vi "Auto Control.vi"   [LabVIEW 2018]
uses:
  <vilib>/Rock Robotics/Network Tables/NT Write String Array.vi
  SubSystems/Drive Train/Drive Train Global.vi
  Robot Global Data.vi
  SubSystems/Hatch Panel Intake/Hatch Panel Intake Global.vi
  SubSystems/Lift/Lift Global.vi
  SubSystems/Cargo Intake/Cargo Intake Global.vi
types:
  T1 = cluster{"X PID":cluster{"proportional gain (Kc)":dbl, "integral time (Ti, min)":dbl, "derivative time (Td, min)":dbl}, "Y PID":cluster{"proportional gain (Kc)":dbl, "integral time (Ti, min)":dbl, "derivative time (Td, min)":dbl}, "Z PID":cluster{"proportional gain (Kc)":dbl, "integral time (Ti, min)":dbl, "derivative time (Td, min)":dbl}}
  T2 = enum16{"Hatch Panel Zone 1", "Hatch Panel Zone 2", "Hatch Panel Zone 3", "Cargo Zone 1", "Cargo Zone 2", "Cargo Zone 3", "Cargo Ship Zone"}
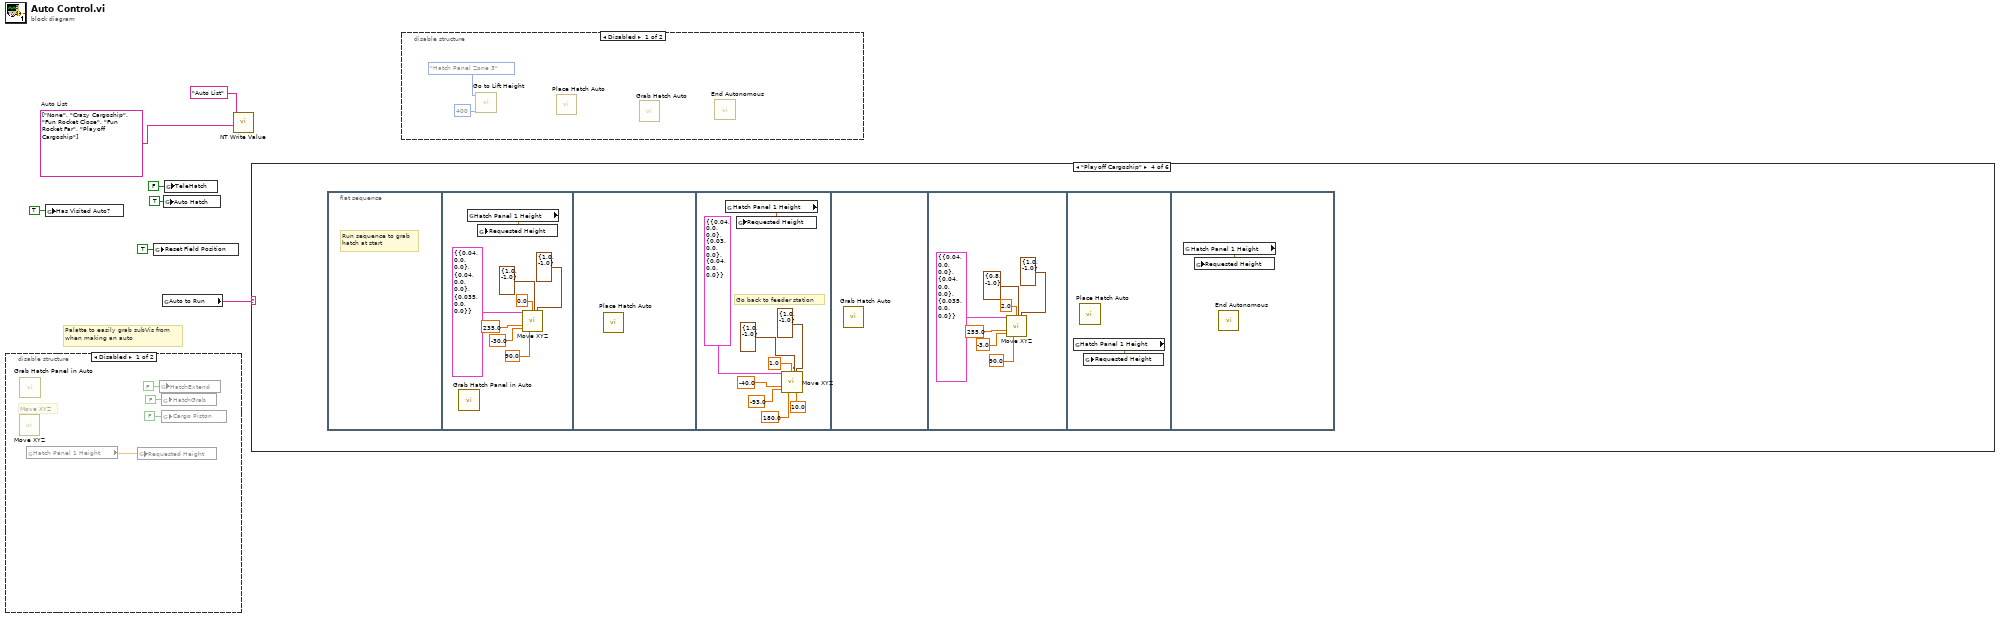
[diagram p0: block diagram]
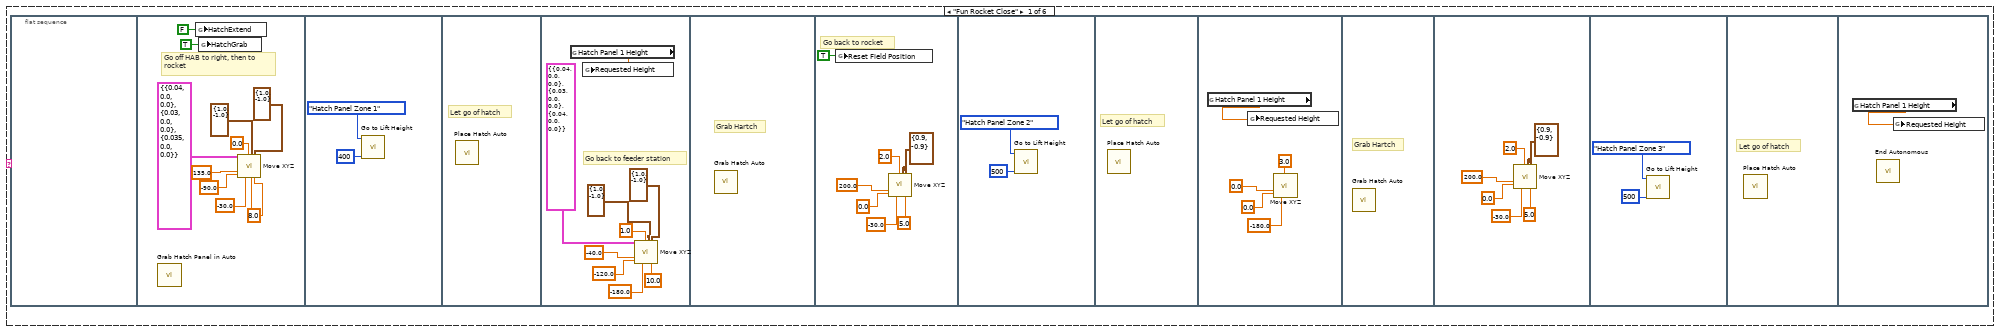
[diagram p4: hidden frame]
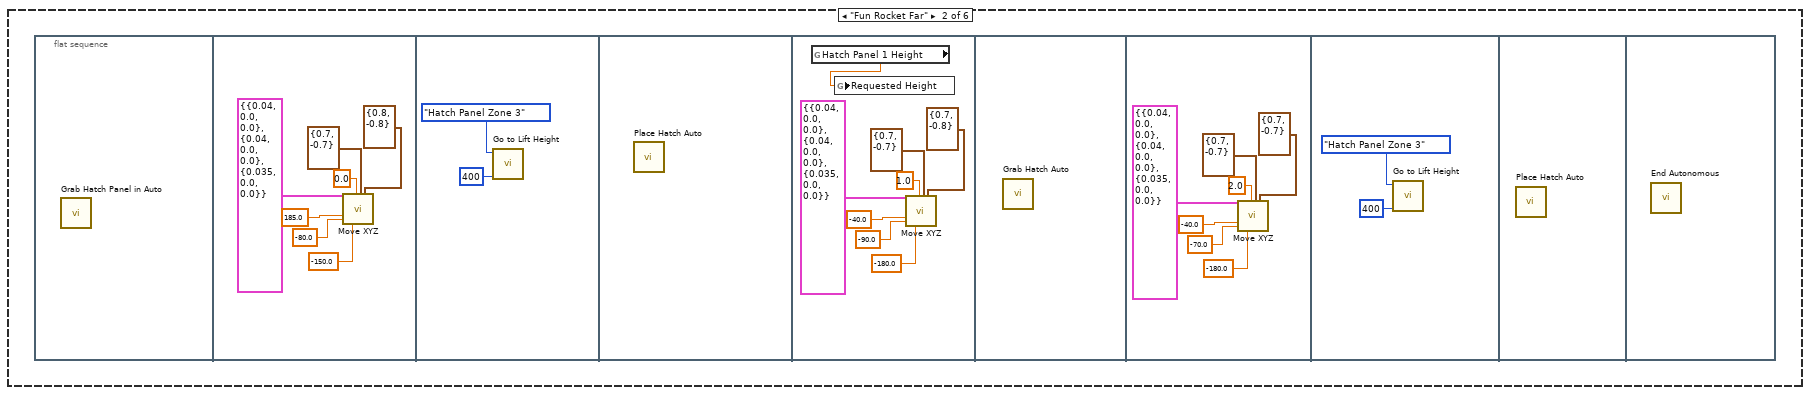
[diagram p5: hidden frame]
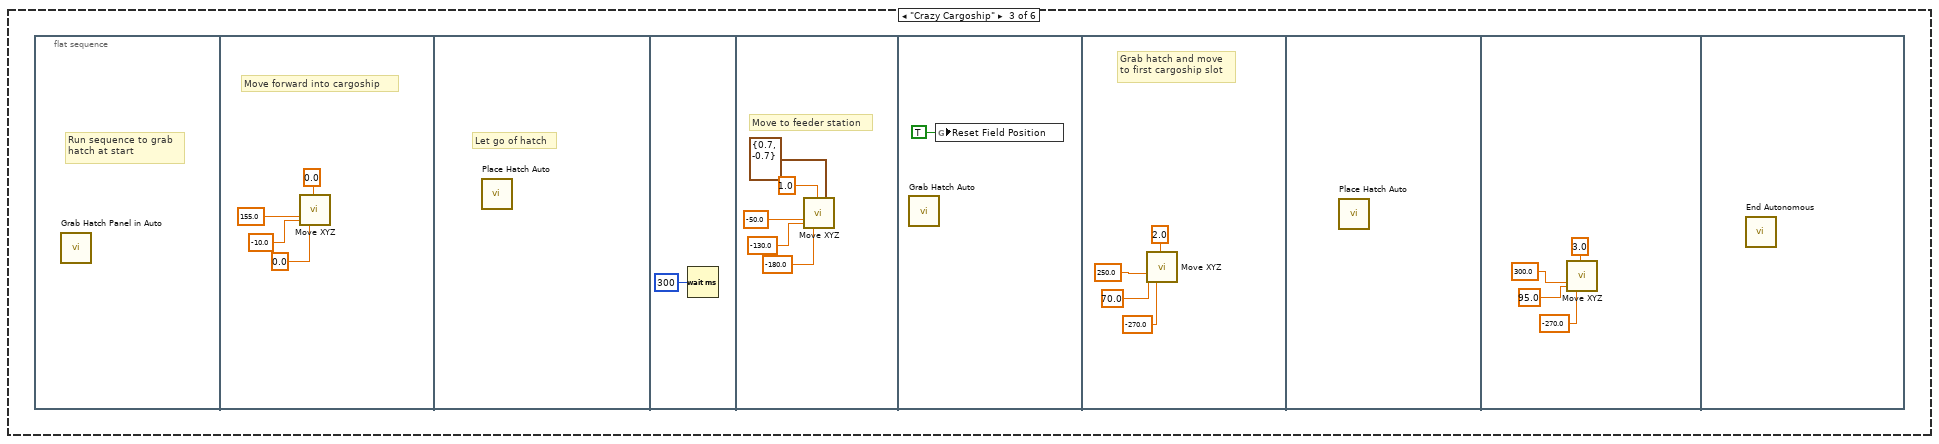
[diagram p6: hidden frame]
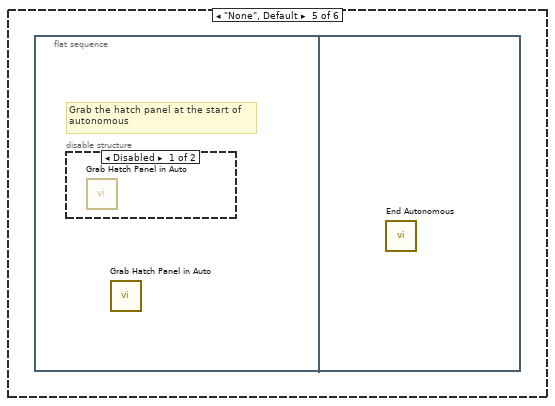
[diagram p7: hidden frame]
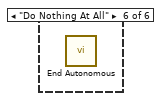
[diagram p9: hidden frame]
diagram:
  w6 = string[] ["None", "Crazy Cargoship", "Fun Rocket Close", "Fun Rocket Far", "Playoff Cargoship"]  # Auto List
  # "Palatte to easily grab subVis from\nwhen making an auto"
  n1 = disable-structure shown="Disabled" {
    frame Disabled {
      # "Move XYZ"
      n2 = call "Move XYZ.vi"() -> ()  [unwired: 28 in]
      n3 = call "Grab Hatch Panel in Auto.vi"() -> ()  [unwired: 12 in]
      n4 = global read "Lift Global.vi" "Hatch Panel 1 Height"() -> (w11:dbl)
      n5 = global write "Lift Global.vi" "Requested Height"(w11) -> ()
      n6 = global write "Hatch Panel Intake Global.vi" "HatchExtend"(FALSE ("HatchExtend")) -> ()
      n7 = global write "Hatch Panel Intake Global.vi" "HatchGrab"(FALSE ("HatchGrab")) -> ()
      n8 = global write "Cargo Intake Global.vi" "Cargo Piston"(FALSE ("Cargo Piston")) -> ()
    }
    frame Enabled {
    }
  }
  n9 = global write "Robot Global Data.vi" "Has Visited Auto?"(TRUE ("Has Visited Auto?")) -> ()
  n10 = global write "Drive Train Global.vi" "Reset Field Position"(TRUE ("Reset Field Position")) -> ()
  n11 = global read "Robot Global Data.vi" "Auto to Run"() -> (w5:string)
  n12 = global write "Hatch Panel Intake Global.vi" "Auto Hatch"(TRUE ("TeleHatch")) -> ()
  n13 = global write "Hatch Panel Intake Global.vi" "TeleHatch"(FALSE ("TeleHatch")) -> ()
  n14 = call-poly <vilib>:"NT Write Value.vi"("String Array"=w6, "Name"="Auto List") -> ()  [unwired: 9 in, 1 out]
  n15 = case shown="\"Playoff Cargoship\"" w5 {
    frame "Fun Rocket Close" {
      n16 = flat-sequence {
        frame #0 {
        }
        frame #1 {
          w15 = 8.0 ("X Stop Threshold")
          # "Go off HAB to right, then to\nrocket"
          n17 = call "Grab Hatch Panel in Auto.vi"() -> ()  [unwired: 12 in]
          n18 = global write "Hatch Panel Intake Global.vi" "HatchExtend"(FALSE ("HatchExtend")) -> ()
          n19 = global write "Hatch Panel Intake Global.vi" "HatchGrab"(TRUE ("HatchGrab")) -> ()
          n20 = call "Move XYZ.vi"("PID Gains In"=T1 {"X PID"={"proportional gain (Kc)"=0.04, "integral time (Ti, min)"=0.0, "derivative time (Td, min)"=0.0}, "Y PID"={"proportional gain (Kc)"=0.03, "integral time (Ti, min)"=0.0, "derivative time (Td, min)"=0.0}, "Z PID"={"proportional gain (Kc)"=0.035, "integral time (Ti, min)"=0.0, "derivative time (Td, min)"=0.0}}, "Y Target"=135.0, "X Target"=-90.0, "Gyro Target"=-30.0, "Movement"=0.0, "X Output Range"=cluster{"output high":dbl, "output low":dbl} {"output high"=1.0, "output low"=-1.0}, "X Stop Threshold"=w15, "Y Output Range"=cluster{"output high":dbl, "output low":dbl} {"output high"=1.0, "output low"=-1.0} ("X Output Range"), "Y Stop Threshold"=w15) -> ()  [unwired: 19 in]
        }
        frame #2 {
          n21 = call "Go to Lift Height.vi"("Time to Settle"=u32 400, "Lift Height to Go To"=T2."Hatch Panel Zone 1" ("y")) -> ()  [unwired: 10 in]
        }
        frame #3 {
          # "Let go of hatch"
          n22 = call "Place Hatch Auto.vi"() -> ()  [unwired: 12 in]
        }
        frame #4 {
          # "Go back to feeder station"
          n23 = global read "Lift Global.vi" "Hatch Panel 1 Height"() -> (w24:dbl)
          n24 = global write "Lift Global.vi" "Requested Height"(w24) -> ()
          n25 = call "Move XYZ.vi"("PID Gains In"=T1 {"X PID"={"proportional gain (Kc)"=0.04, "integral time (Ti, min)"=0.0, "derivative time (Td, min)"=0.0}, "Y PID"={"proportional gain (Kc)"=0.03, "integral time (Ti, min)"=0.0, "derivative time (Td, min)"=0.0}, "Z PID"={"proportional gain (Kc)"=0.04, "integral time (Ti, min)"=0.0, "derivative time (Td, min)"=0.0}}, "Y Target"=-40.0, "X Target"=-120.0, "Gyro Target"=-180.0, "Movement"=1.0, "X Output Range"=cluster{"output high":dbl, "output low":dbl} {"output high"=1.0, "output low"=-1.0}, "Y Output Range"=cluster{"output high":dbl, "output low":dbl} {"output high"=1.0, "output low"=-1.0} ("X Output Range"), "Y Stop Threshold"=10.0) -> ()  [unwired: 20 in]
        }
        frame #5 {
          # "Grab Hartch"
          n26 = call "Grab Hatch Auto.vi"() -> ()  [unwired: 12 in]
        }
        frame #6 {
          w33 = cluster{"output high":dbl, "output low":dbl} {"output high"=0.9, "output low"=-0.9} ("Y Output Range")
          # "Go back to rocket"
          n27 = global write "Drive Train Global.vi" "Reset Field Position"(TRUE ("Reset Field Position")) -> ()
          n28 = call "Move XYZ.vi"("Y Target"=200.0, "X Target"=0.0, "Gyro Target"=-30.0, "Movement"=2.0, "X Output Range"=w33, "Y Output Range"=w33, "Y Stop Threshold"=5.0) -> ()  [unwired: 21 in]
        }
        frame #7 {
          n29 = call "Go to Lift Height.vi"("Time to Settle"=u32 500, "Lift Height to Go To"=T2."Hatch Panel Zone 2" ("y")) -> ()  [unwired: 10 in]
        }
        frame #8 {
          # "Let go of hatch"
          n30 = call "Place Hatch Auto.vi"() -> ()  [unwired: 12 in]
        }
        frame #9 {
          n31 = global read "Lift Global.vi" "Hatch Panel 1 Height"() -> (w46:dbl)
          n32 = global write "Lift Global.vi" "Requested Height"(w46) -> ()
          n33 = call "Move XYZ.vi"("Y Target"=0.0, "X Target"=0.0, "Gyro Target"=-180.0, "Movement"=3.0) -> ()  [unwired: 24 in]
        }
        frame #10 {
          # "Grab Hartch"
          n34 = call "Grab Hatch Auto.vi"() -> ()  [unwired: 12 in]
        }
        frame #11 {
          w47 = cluster{"output high":dbl, "output low":dbl} {"output high"=0.9, "output low"=-0.9} ("Y Output Range")
          n35 = call "Move XYZ.vi"("Y Target"=200.0, "X Target"=0.0, "Gyro Target"=-30.0, "Movement"=2.0, "X Output Range"=w47, "Y Output Range"=w47, "Y Stop Threshold"=5.0) -> ()  [unwired: 21 in]
        }
        frame #12 {
          n36 = call "Go to Lift Height.vi"("Time to Settle"=u32 500, "Lift Height to Go To"=T2."Hatch Panel Zone 3" ("y")) -> ()  [unwired: 10 in]
        }
        frame #13 {
          # "Let go of hatch"
          n37 = call "Place Hatch Auto.vi"() -> ()  [unwired: 12 in]
        }
        frame #14 {
          n38 = global read "Lift Global.vi" "Hatch Panel 1 Height"() -> (w55:dbl)
          n39 = call "End Autonomous.vi"() -> ()  [unwired: 12 in]
          n40 = global write "Lift Global.vi" "Requested Height"(w55) -> ()
        }
      }
    }
    frame "Fun Rocket Far" {
      n41 = flat-sequence {
        frame #0 {
          n42 = call "Grab Hatch Panel in Auto.vi"() -> ()  [unwired: 12 in]
        }
        frame #1 {
          n43 = call "Move XYZ.vi"("PID Gains In"=T1 {"X PID"={"proportional gain (Kc)"=0.04, "integral time (Ti, min)"=0.0, "derivative time (Td, min)"=0.0}, "Y PID"={"proportional gain (Kc)"=0.04, "integral time (Ti, min)"=0.0, "derivative time (Td, min)"=0.0}, "Z PID"={"proportional gain (Kc)"=0.035, "integral time (Ti, min)"=0.0, "derivative time (Td, min)"=0.0}}, "Y Target"=185.0, "X Target"=-80.0, "Gyro Target"=-150.0, "Movement"=0.0, "X Output Range"=cluster{"output high":dbl, "output low":dbl} {"output high"=0.7, "output low"=-0.7}, "Y Output Range"=cluster{"output high":dbl, "output low":dbl} {"output high"=0.8, "output low"=-0.8} ("X Output Range")) -> ()  [unwired: 21 in]
        }
        frame #2 {
          n44 = call "Go to Lift Height.vi"("Time to Settle"=u32 400, "Lift Height to Go To"=T2."Hatch Panel Zone 3" ("y")) -> ()  [unwired: 10 in]
        }
        frame #3 {
          n45 = call "Place Hatch Auto.vi"() -> ()  [unwired: 12 in]
        }
        frame #4 {
          n46 = global read "Lift Global.vi" "Hatch Panel 1 Height"() -> (w65:dbl)
          n47 = global write "Lift Global.vi" "Requested Height"(w65) -> ()
          n48 = call "Move XYZ.vi"("PID Gains In"=T1 {"X PID"={"proportional gain (Kc)"=0.04, "integral time (Ti, min)"=0.0, "derivative time (Td, min)"=0.0}, "Y PID"={"proportional gain (Kc)"=0.04, "integral time (Ti, min)"=0.0, "derivative time (Td, min)"=0.0}, "Z PID"={"proportional gain (Kc)"=0.035, "integral time (Ti, min)"=0.0, "derivative time (Td, min)"=0.0}}, "Y Target"=-40.0, "X Target"=-90.0, "Gyro Target"=-180.0, "Movement"=1.0, "X Output Range"=cluster{"output high":dbl, "output low":dbl} {"output high"=0.7, "output low"=-0.7}, "Y Output Range"=cluster{"output high":dbl, "output low":dbl} {"output high"=0.7, "output low"=-0.8} ("X Output Range")) -> ()  [unwired: 21 in]
        }
        frame #5 {
          n49 = call "Grab Hatch Auto.vi"() -> ()  [unwired: 12 in]
        }
        frame #6 {
          n50 = call "Move XYZ.vi"("PID Gains In"=T1 {"X PID"={"proportional gain (Kc)"=0.04, "integral time (Ti, min)"=0.0, "derivative time (Td, min)"=0.0}, "Y PID"={"proportional gain (Kc)"=0.04, "integral time (Ti, min)"=0.0, "derivative time (Td, min)"=0.0}, "Z PID"={"proportional gain (Kc)"=0.035, "integral time (Ti, min)"=0.0, "derivative time (Td, min)"=0.0}}, "Y Target"=-40.0, "X Target"=-70.0, "Gyro Target"=-180.0, "Movement"=2.0, "X Output Range"=cluster{"output high":dbl, "output low":dbl} {"output high"=0.7, "output low"=-0.7}, "Y Output Range"=cluster{"output high":dbl, "output low":dbl} {"output high"=0.7, "output low"=-0.7} ("X Output Range")) -> ()  [unwired: 21 in]
        }
        frame #7 {
          n51 = call "Go to Lift Height.vi"("Time to Settle"=u32 400, "Lift Height to Go To"=T2."Hatch Panel Zone 3" ("y")) -> ()  [unwired: 10 in]
        }
        frame #8 {
          n52 = call "Place Hatch Auto.vi"() -> ()  [unwired: 12 in]
        }
        frame #9 {
          n53 = call "End Autonomous.vi"() -> ()  [unwired: 12 in]
        }
      }
    }
    frame "Crazy Cargoship" {
      n54 = flat-sequence {
        frame #0 {
          # "Run sequence to grab\nhatch at start"
          n55 = call "Grab Hatch Panel in Auto.vi"() -> ()  [unwired: 12 in]
        }
        frame #1 {
          # "Move forward into cargoship"
          n56 = call "Move XYZ.vi"("Y Target"=155.0, "X Target"=-10.0, "Gyro Target"=0.0, "Movement"=0.0) -> ()  [unwired: 24 in]
        }
        frame #2 {
          # "Let go of hatch"
          n57 = call "Place Hatch Auto.vi"() -> ()  [unwired: 12 in]
        }
        frame #3 {
          n58 = Wait (ms)(milliseconds to wait=u32 300) -> ()  [unwired: 1 out]
        }
        frame #4 {
          # "Move to feeder station"
          n59 = call "Move XYZ.vi"("Y Target"=-50.0, "X Target"=-130.0, "Gyro Target"=-180.0, "Movement"=1.0, "Y Output Range"=cluster{"output high":dbl, "output low":dbl} {"output high"=0.7, "output low"=-0.7}) -> ()  [unwired: 23 in]
        }
        frame #5 {
          n60 = call "Grab Hatch Auto.vi"() -> ()  [unwired: 12 in]
          n61 = global write "Drive Train Global.vi" "Reset Field Position"(TRUE ("Reset Field Position")) -> ()
        }
        frame #6 {
          # "Grab hatch and move\nto first cargoship slot"
          n62 = call "Move XYZ.vi"("Y Target"=250.0, "X Target"=70.0, "Gyro Target"=-270.0, "Movement"=2.0) -> ()  [unwired: 24 in]
        }
        frame #7 {
          n63 = call "Place Hatch Auto.vi"() -> ()  [unwired: 12 in]
        }
        frame #8 {
          n64 = call "Move XYZ.vi"("Y Target"=300.0, "X Target"=95.0, "Gyro Target"=-270.0, "Movement"=3.0) -> ()  [unwired: 24 in]
        }
        frame #9 {
          n65 = call "End Autonomous.vi"() -> ()  [unwired: 12 in]
        }
      }
    }
    frame "Playoff Cargoship" {
      n66 = flat-sequence {
        frame #0 {
          # "Run sequence to grab\nhatch at start"
        }
        frame #1 {
          n67 = call "Grab Hatch Panel in Auto.vi"() -> ()  [unwired: 12 in]
          n68 = global read "Lift Global.vi" "Hatch Panel 1 Height"() -> (w101:dbl)
          n69 = global write "Lift Global.vi" "Requested Height"(w101) -> ()
          n70 = call "Move XYZ.vi"("PID Gains In"=T1 {"X PID"={"proportional gain (Kc)"=0.04, "integral time (Ti, min)"=0.0, "derivative time (Td, min)"=0.0}, "Y PID"={"proportional gain (Kc)"=0.04, "integral time (Ti, min)"=0.0, "derivative time (Td, min)"=0.0}, "Z PID"={"proportional gain (Kc)"=0.035, "integral time (Ti, min)"=0.0, "derivative time (Td, min)"=0.0}}, "Y Target"=235.0, "X Target"=-30.0, "Gyro Target"=90.0, "Movement"=0.0, "X Output Range"=cluster{"output high":dbl, "output low":dbl} {"output high"=1.0, "output low"=-1.0}, "Y Output Range"=cluster{"output high":dbl, "output low":dbl} {"output high"=1.0, "output low"=-1.0} ("X Output Range")) -> ()  [unwired: 21 in]
        }
        frame #2 {
          n71 = call "Place Hatch Auto.vi"() -> ()  [unwired: 12 in]
        }
        frame #3 {
          # "Go back to feeder station"
          n72 = global read "Lift Global.vi" "Hatch Panel 1 Height"() -> (w109:dbl)
          n73 = global write "Lift Global.vi" "Requested Height"(w109) -> ()
          n74 = call "Move XYZ.vi"("PID Gains In"=T1 {"X PID"={"proportional gain (Kc)"=0.04, "integral time (Ti, min)"=0.0, "derivative time (Td, min)"=0.0}, "Y PID"={"proportional gain (Kc)"=0.03, "integral time (Ti, min)"=0.0, "derivative time (Td, min)"=0.0}, "Z PID"={"proportional gain (Kc)"=0.04, "integral time (Ti, min)"=0.0, "derivative time (Td, min)"=0.0}}, "Y Target"=-40.0, "X Target"=-93.0, "Gyro Target"=180.0, "Movement"=1.0, "X Output Range"=cluster{"output high":dbl, "output low":dbl} {"output high"=1.0, "output low"=-1.0}, "Y Output Range"=cluster{"output high":dbl, "output low":dbl} {"output high"=1.0, "output low"=-1.0} ("X Output Range"), "Y Stop Threshold"=10.0) -> ()  [unwired: 20 in]
        }
        frame #4 {
          n75 = call "Grab Hatch Auto.vi"() -> ()  [unwired: 12 in]
        }
        frame #5 {
          n76 = call "Move XYZ.vi"("PID Gains In"=T1 {"X PID"={"proportional gain (Kc)"=0.04, "integral time (Ti, min)"=0.0, "derivative time (Td, min)"=0.0}, "Y PID"={"proportional gain (Kc)"=0.04, "integral time (Ti, min)"=0.0, "derivative time (Td, min)"=0.0}, "Z PID"={"proportional gain (Kc)"=0.035, "integral time (Ti, min)"=0.0, "derivative time (Td, min)"=0.0}}, "Y Target"=255.0, "X Target"=-3.0, "Gyro Target"=90.0, "Movement"=2.0, "X Output Range"=cluster{"output high":dbl, "output low":dbl} {"output high"=0.8, "output low"=-1.0}, "Y Output Range"=cluster{"output high":dbl, "output low":dbl} {"output high"=1.0, "output low"=-1.0} ("X Output Range")) -> ()  [unwired: 21 in]
        }
        frame #6 {
          n77 = global read "Lift Global.vi" "Hatch Panel 1 Height"() -> (w125:dbl)
          n78 = call "Place Hatch Auto.vi"() -> ()  [unwired: 12 in]
          n79 = global write "Lift Global.vi" "Requested Height"(w125) -> ()
        }
        frame #7 {
          n80 = global read "Lift Global.vi" "Hatch Panel 1 Height"() -> (w126:dbl)
          n81 = global write "Lift Global.vi" "Requested Height"(w126) -> ()
          n82 = call "End Autonomous.vi"() -> ()  [unwired: 12 in]
        }
      }
    }
    frame "None", Default {
      n83 = flat-sequence {
        frame #0 {
          # "Grab the hatch panel at the start of \nautonomous"
          n84 = disable-structure shown="Disabled" {
            frame Disabled {
              n85 = call "Grab Hatch Panel in Auto.vi"() -> ()  [unwired: 12 in]
            }
            frame Enabled {
            }
          }
          n86 = call "Grab Hatch Panel in Auto.vi"() -> ()  [unwired: 12 in]
        }
        frame #1 {
          n87 = call "End Autonomous.vi"() -> ()  [unwired: 12 in]
        }
      }
    }
    frame "Do Nothing At All" {
      n88 = call "End Autonomous.vi"() -> ()  [unwired: 12 in]
    }
  }
  n89 = disable-structure shown="Disabled" {
    frame Disabled {
      n90 = call "Go to Lift Height.vi"("Time to Settle"=u32 400, "Lift Height to Go To"=T2."Hatch Panel Zone 3" ("y")) -> ()  [unwired: 10 in]
      n91 = call "Place Hatch Auto.vi"() -> ()  [unwired: 12 in]
      n92 = call "Grab Hatch Auto.vi"() -> ()  [unwired: 12 in]
      n93 = call "End Autonomous.vi"() -> ()  [unwired: 12 in]
    }
    frame Enabled {
    }
  }
